vi "stepper-4.vi"() -> ()   [LabVIEW 2018]
uses:
  <vilib>/Platform/TimedLoop/XDataNode/timing_clust.ctl
  <vilib>/Platform/TimedLoop/XDataNode/nitl_modes.ctl
  <vilib>/Platform/TimedLoop/XDataNode/wakeup.ctl
  <vilib>/FPGAPlugInAG/myRIO-1900/niLvFpga_Open_myRIO-1900.vi
  <vilib>/rvi/interface/common/dynamic/niFpgaDynamicAddResources.vi
  <vilib>/Utility/error.llb/Error Cluster From Error Code.vi
  <vilib>/rvi/errors/niLvFpgaAdjustHostInterfaceError.vi
  <vilib>/rvi/interface/nirviOpenFPGA/nirviOpenFPGA.xnode
  FPGA Bitfiles/Dentalrobot_FPGATarget_1DIOBoardTestFPG_Hns6xIf0z6s.lvbitx
  FPGA/FPGA_Dental robot.vi
  <vilib>/rvi/interface/nirviReadWriteControl/nirviReadWriteControl.xnode
  <vilib>/Platform/TimedLoop/XDataNode/XDataNode.xnode
  <vilib>/Platform/TimedLoop/XDataNode/XDNodeRunTimeDep.lvlib
  <vilib>/rvi/interface/Simulation/niFpgaSimulationCallBeginRW.vi
  NiFpgaLv.dll
panel:
  in  "STBY4":bool
  in  "ENA4":bool
  in  "CH4 DC":fxp<+,32,0>
  out "Cluster":T1
  in  "Step":u32 step=400
  in  "steps / round":u32=200
  in  "rpm":u32=200 min=10 max=1000 step=10
  in  "Dir":bool
  in  "stop":bool
  # "max speed : ~400rpm"
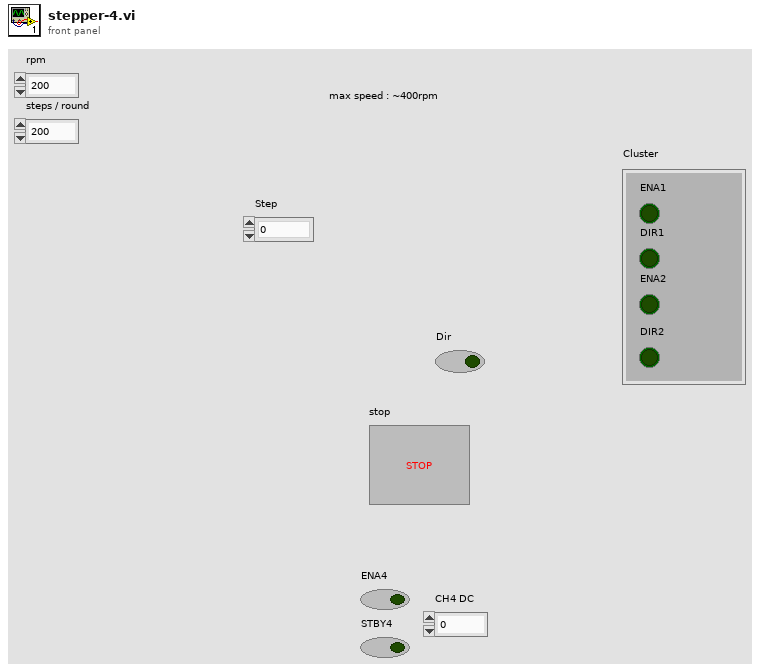
[diagram p1: front panel]
types:
  T1 = cluster{"ENA1":bool, "DIR1":bool, "ENA2":bool, "DIR2":bool}
  T2 = typedef "XDNodeRunTimeDep.lvlib/timing_clust.ctl" = cluster{"Expected End [f-1]":u64, "Actual End [f-1]":u64, "Finished Late? [f-1]":bool, "Expected End [i-1]":u64, "Actual End [i-1]":u64, "Finished Late? [i-1]":bool, "Expected Start [i]":u64, "Actual Start [i]":u64, "Expected Start [f]":u64, "Actual Start [f]":u64, "Source Name":string, "Structure Name":string, "Period":i64, "Deadline":i64, "Offset":i64, "Start":i64, "Priority":i32, "Timeout":i32, "Mode":T3, "Wakeup Reason":T4, "Error":errorcluster, "Source Type":string, "Secondary Source Type":string, "Global End Time":u64, "Global Start Time":u64, "Frame Duration":u64, "Iteration Duration":u64, "Assigned CPU":i32, "I/O Scan Engine Mode":u32}
  T3 = typedef "XDNodeRunTimeDep.lvlib/nitl_modes.ctl" = enum32{"No Change", "Process missed periods, maintain original phase", "Discard missed periods, maintain original phase", "Process missed periods, ignore original phase", "Discard missed periods, ignore original phase"}
  T4 = typedef "XDNodeRunTimeDep.lvlib/wakeup.ctl" = enum32{"Normal", "Aborted", "Asynchronous wakeup", "Timing source error", "Timed loop error", "Timeout"}
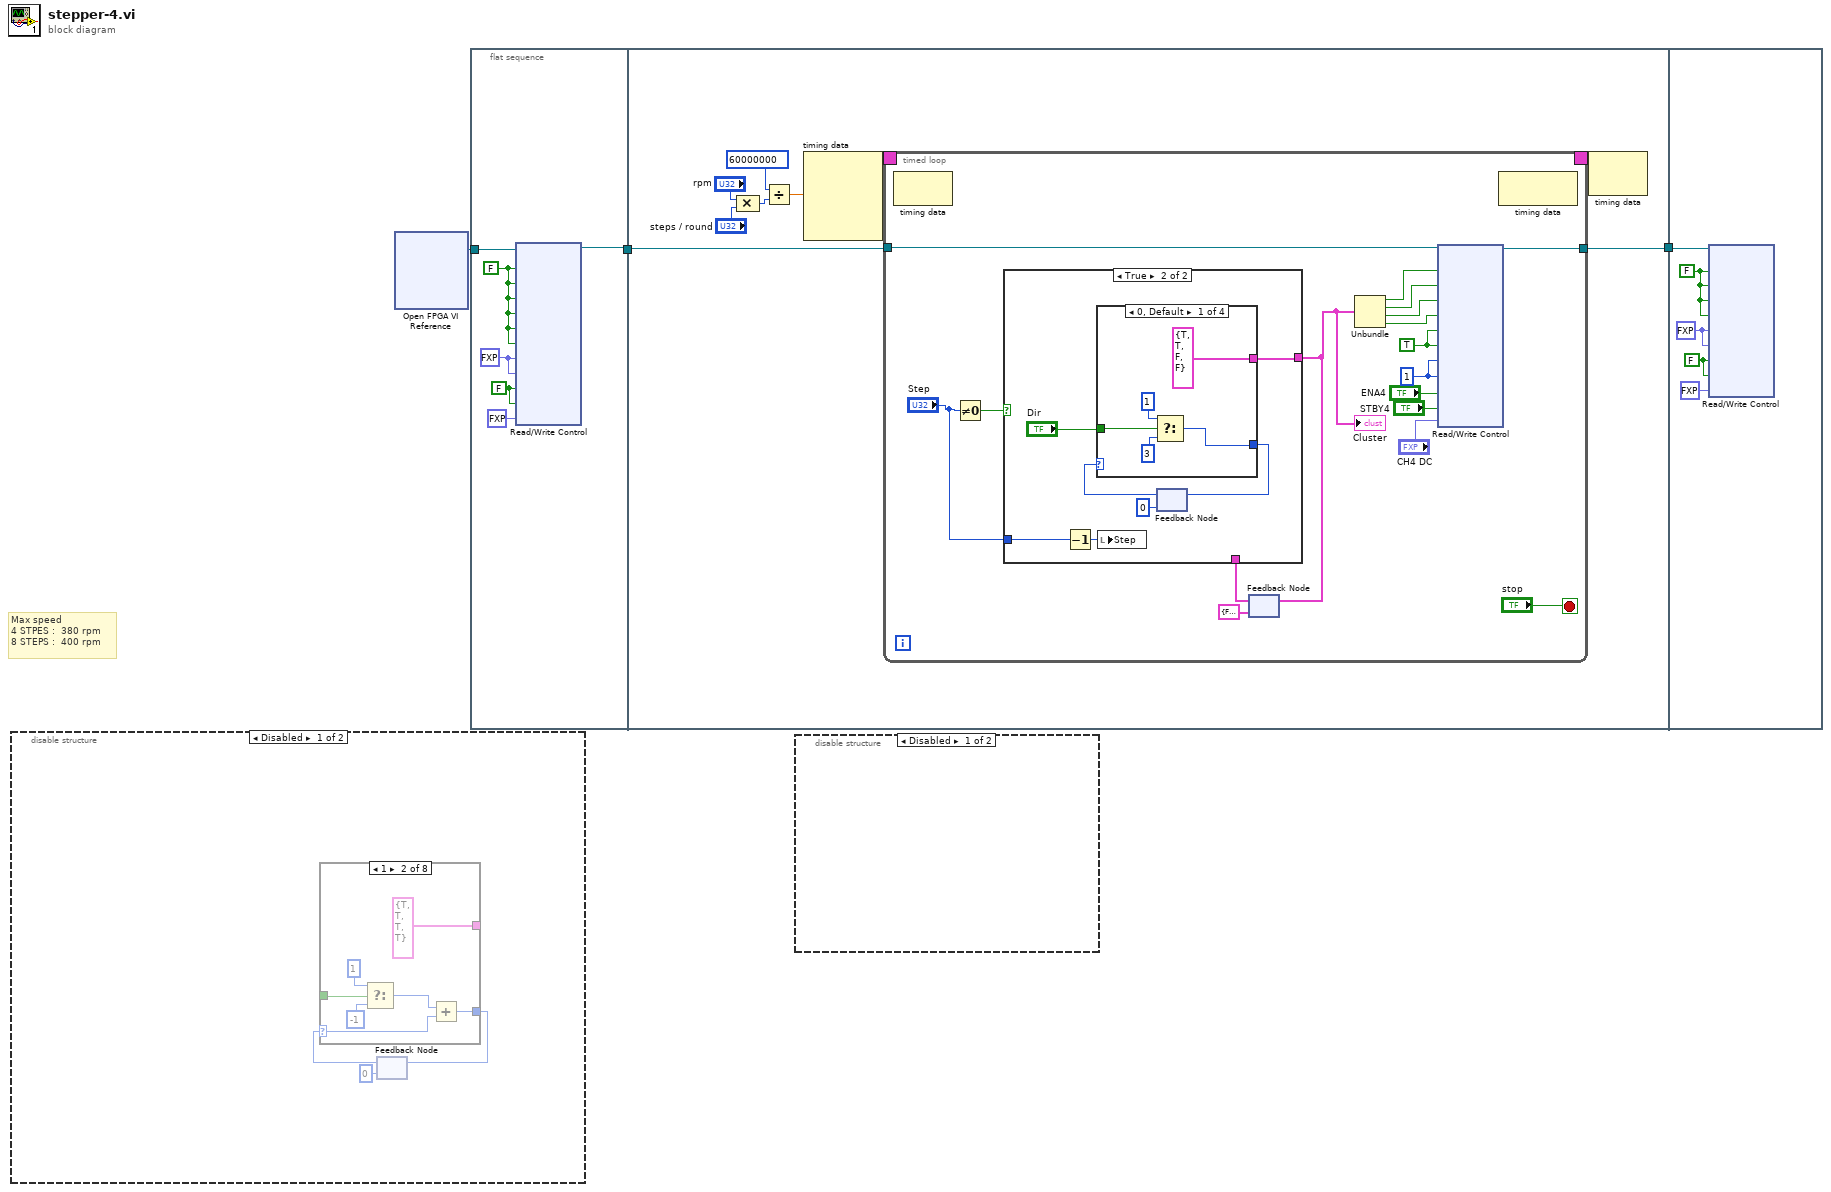
[diagram p0: block diagram]
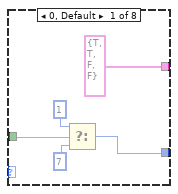
[diagram p3: hidden frame]
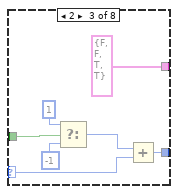
[diagram p4: hidden frame]
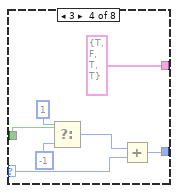
[diagram p5: hidden frame]
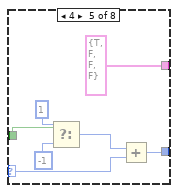
[diagram p6: hidden frame]
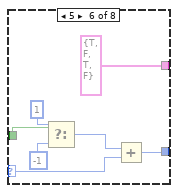
[diagram p7: hidden frame]
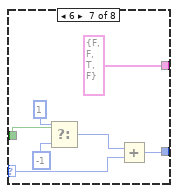
[diagram p8: hidden frame]
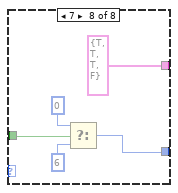
[diagram p9: hidden frame]
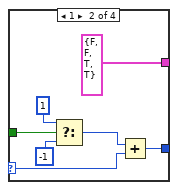
[diagram p12: hidden frame]
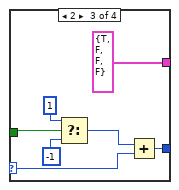
[diagram p13: hidden frame]
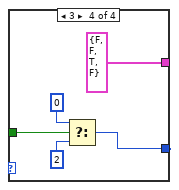
[diagram p14: hidden frame]
diagram:
  # "Max speed\n4 STPES :  380 rpm\n8 STEPS :  400 rpm"
  n1 = disable-structure shown="Disabled" {
    frame Disabled {
      n2 = feedback #1(0) -> (w5:u32)
      n3 = case shown="1" w5 {
        selector: w5 -> [_ w18 w25 w28 w34 w41 w48 _]
        tunnel: [w9 w19 w26 w27 w35 w43 w51 w55] -> w6
        tunnel: [w12 w15 w22 w29 w36 w42 w49 w56] -> w4
        tunnel: [cluster{bool, bool, bool, bool} {TRUE, TRUE, FALSE, FALSE} cluster{bool, bool, bool, bool} {TRUE, TRUE, TRUE, TRUE} cluster{bool, bool, bool, bool} {FALSE, FALSE, TRUE, TRUE} cluster{bool, bool, bool, bool} {TRUE, FALSE, TRUE, TRUE} cluster{bool, bool, bool, bool} {TRUE, FALSE, FALSE, FALSE} cluster{bool, bool, bool, bool} {TRUE, FALSE, TRUE, FALSE} cluster{bool, bool, bool, bool} {FALSE, FALSE, TRUE, FALSE} cluster{bool, bool, bool, bool} {TRUE, TRUE, TRUE, FALSE}] -> _
        frame 0, Default {
          n4 = Select(t=1, s=w12, f=7) -> (s? t:f=w9:i32)
        }
        frame 1 {
          n5 = Select(t=1, s=w15, f=-1) -> (s? t:f=w14:i32)
          n6 = Add(x=w14, y=w18) -> (x+y=w19:u32)
        }
        frame 2 {
          n7 = Select(t=1, s=w22, f=-1) -> (s? t:f=w21:i32)
          n8 = Add(x=w21, y=w25) -> (x+y=w26:u32)
        }
        frame 3 {
          n9 = Select(t=1, s=w29, f=-1) -> (s? t:f=w30:i32)
          n10 = Add(x=w30, y=w28) -> (x+y=w27:u32)
        }
        frame 4 {
          n11 = Select(t=1, s=w36, f=-1) -> (s? t:f=w38:i32)
          n12 = Add(x=w38, y=w34) -> (x+y=w35:u32)
        }
        frame 5 {
          n13 = Select(t=1, s=w42, f=-1) -> (s? t:f=w45:i32)
          n14 = Add(x=w45, y=w41) -> (x+y=w43:u32)
        }
        frame 6 {
          n15 = Select(t=1, s=w49, f=-1) -> (s? t:f=w52:i32)
          n16 = Add(x=w52, y=w48) -> (x+y=w51:u32)
        }
        frame 7 {
          n17 = Select(t=0, s=w56, f=6) -> (s? t:f=w55:i32)
        }
      }
      n18 = feedback-in #1(w6) -> ()
    }
    frame Enabled {
    }
  }
  n19 = xnode "Open FPGA VI Reference"() -> ("FPGA VI Reference Out"=w1:refnum<k20>)  [unwired: 2 in, 1 out]
  n20 = flat-sequence {
    tunnel: [w64] -> w2
    tunnel: w1 -> [w62]
    tunnel: [w74] -> w3
    tunnel: w2 -> [w73]
    tunnel: w3 -> [w134]
    frame #0 {
      w60 = FALSE ("ENA4")
      w63 = fxp<+,32,0> 0.0 ("CH1 DC")
      w65 = FALSE ("ENA1")
      n21 = xnode "Read/Write Control"("FPGA VI Reference In"=w62, "ENA1"=w65, "STBY1"=w65, "DIR1"=w65, "ENA2"=w65, "STBY2"=w65, "DIR2"=w65, "CH1 DC"=w63, "CH2 DC"=w63, "ENA4"=w60, "STBY4"=w60, "CH4 DC"=fxp<+,32,0> 0.0) -> ("FPGA VI Reference Out"=w64:refnum<k20>)  [unwired: 1 in, 1 out]
    }
    frame #1 {
      n22 = Compound Arithmetic op=MULTIPLY("rpm", "steps / round") -> (w68:u32)
      n23 = Divide(x=i64 60000000, y=w68) -> (x/y=w66:dbl)
      n24 = node-c288(w66) -> (w72:T2)  [unwired: 3 in]
      n25 = timed-loop {
        timing: w72 -> [_]
        timing-out: [_] -> w71
        tunnel: [w91] -> w74
        tunnel: w73 -> [w90]
        stop <- "stop" stop-if-true
        w84 = 1 ("CH1 DC")
        w88 = TRUE ("STBY1")
        n26 = node-c288() -> ()  [unwired: 1 in, 1 out]
        n27 = Not Equal To 0?(x="Step") -> (x != 0?=w83:bool)
        n28 = feedback #2(cluster{bool, bool, bool, bool} {FALSE, FALSE, FALSE, FALSE}) -> (w81:cluster{bool, bool, bool, bool})
        n29 = case shown="True" w83 {
          tunnel: [w92 w94] -> w79
          tunnel: "Step" -> [_ w98]
          tunnel: w81 -> [w92 _]
          frame False {
          }
          frame True {
            n30 = Decrement(x=w98) -> (x-1=w99:u32)
            n31 = local write "Step"(w99) -> ()
            n32 = feedback #3(0) -> (w97:u32)
            n33 = case shown="0, Default" w97 {
              selector: w97 -> [_ w110 w117 _]
              tunnel: [w101 w111 w118 w120] -> w95
              tunnel: "Dir" -> [w104 w107 w114 w121]
              tunnel: [cluster{bool, bool, bool, bool} {TRUE, TRUE, FALSE, FALSE} cluster{bool, bool, bool, bool} {FALSE, FALSE, TRUE, TRUE} cluster{bool, bool, bool, bool} {TRUE, FALSE, FALSE, FALSE} cluster{bool, bool, bool, bool} {FALSE, FALSE, TRUE, FALSE}] -> w94
              frame 0, Default {
                n34 = Select(t=1, s=w104, f=3) -> (s? t:f=w101:i32)
              }
              frame 1 {
                n35 = Select(t=1, s=w107, f=-1) -> (s? t:f=w106:i32)
                n36 = Add(x=w106, y=w110) -> (x+y=w111:u32)
              }
              frame 2 {
                n37 = Select(t=1, s=w114, f=-1) -> (s? t:f=w113:i32)
                n38 = Add(x=w113, y=w117) -> (x+y=w118:u32)
              }
              frame 3 {
                n39 = Select(t=0, s=w121, f=2) -> (s? t:f=w120:i32)
              }
            }
            n40 = feedback-in #3(w95) -> ()
          }
        }
        "Cluster" <- w79
        n41 = feedback-in #2(w79) -> ()
        n42 = Unbundle(w79) -> (w89:bool, w87:bool, w86:bool, w85:bool)
        n43 = xnode "Read/Write Control"("FPGA VI Reference In"=w90, "ENA1"=w89, "DIR1"=w87, "ENA2"=w86, "DIR2"=w85, "STBY1"=w88, "STBY2"=w88, "CH1 DC"=w84, "CH2 DC"=w84, "ENA4"="ENA4", "STBY4"="STBY4", "CH4 DC"="CH4 DC") -> ("FPGA VI Reference Out"=w91:refnum<k20>)  [unwired: 1 in, 1 out]
        n44 = node-c288() -> ()  [unwired: 1 in, 1 out]
      }
      n45 = node-c288(w71) -> ()  [unwired: 1 out]
    }
    frame #2 {
      w131 = FALSE ("ENA4")
      w132 = fxp<+,32,0> 0.0 ("CH1 DC")
      w133 = FALSE ("ENA1")
      n46 = xnode "Read/Write Control"("FPGA VI Reference In"=w134, "ENA1"=w133, "STBY1"=w133, "ENA2"=w133, "STBY2"=w133, "CH1 DC"=w132, "CH2 DC"=w132, "ENA4"=w131, "STBY4"=w131, "CH4 DC"=fxp<+,32,0> 0.0) -> ()  [unwired: 1 in, 2 out]
    }
  }
  n47 = disable-structure shown="Disabled" {
    frame Disabled {
    }
    frame Enabled {
    }
  }
